vi "Part 1.vi"(11 "Input":string) -> (3 "Output":i64)   [LabVIEW 2021]
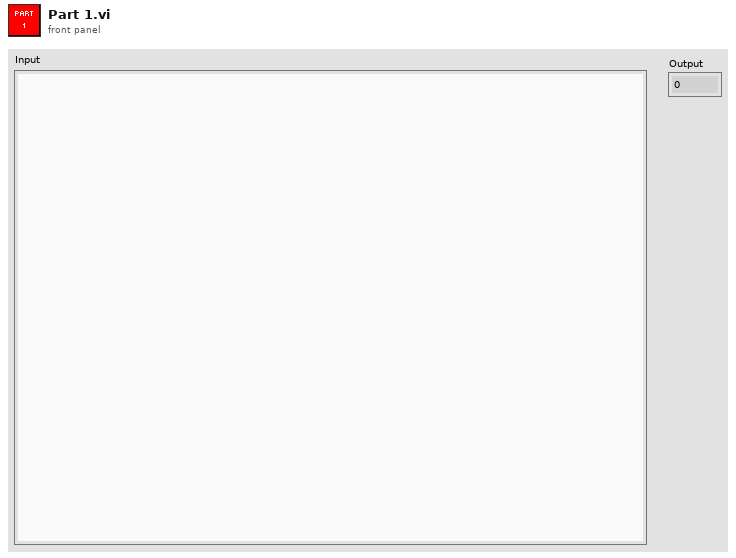
[diagram p1: front panel]
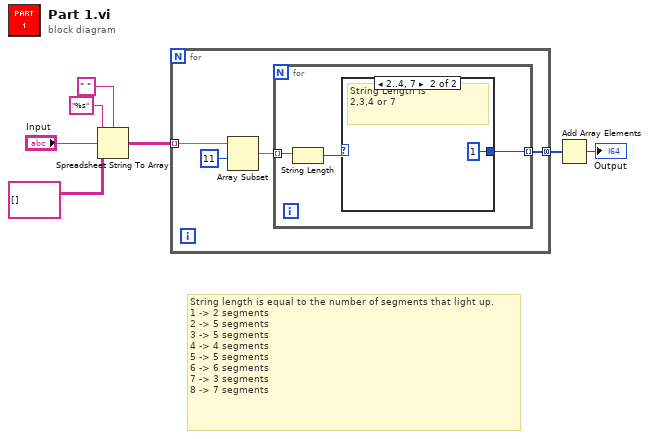
[diagram p0: block diagram]
diagram:
  # "String length is equal to the number of segments that light up.\n1 -> 2 segments\n2 -> 5 segments\n3 -> 5 segments\n4 -> 4 segments\n5 -> 5 segments\n6 -> 6 segments\n7 -> 3 segments\n8 -> 7 segments"
  n1 = Spreadsheet String To Array(delimiter (Tab)=" ", format string="%s", spreadsheet string="Input", array type (2D Dbl)=string[][] []) -> (array=w3:string[][])
  n2 = for {
    tunnel: w3 -> [w11] mode=indexing
    tunnel: [w8] -> w1 mode=concatenating
    n3 = Array Subset(array=w11, index=11) -> (w9:string[])  [unwired: 1 in]
    n4 = for {
      tunnel: w9 -> [w14] mode=indexing
      tunnel: [w12] -> w8 mode=indexing
      n5 = String Length(string=w14) -> (length=w13:i32)
      n6 = case shown="2..4, 7" w13 {
        tunnel: [_ i64 1] -> w12
        frame 0, Default {
        }
        frame 2..4, 7 {
          # "String Length is\n2,3,4 or 7"
        }
      }
    }
  }
  n7 = Add Array Elements(numeric array=w1) -> (sum=→"Output":i64)
